vi "temp_dependent_eV-V_slope.vi"() -> ()   [LabVIEW 2016]
uses:
  <vilib>/Analysis/baseanly.llb/Mean (DBL).vi
  <vilib>/Analysis/NI_AALBase.lvlib
  <vilib>/Analysis/NI_AALPro.lvlib
panel:
  out "1/x ( eV/V)":dbl
  out "intercept":dbl
  out "slope (V/eV)":dbl
  out "XY Graph":cluster{dbl[], dbl[]}(graph)
  out "Array 3":dbl[](array[numeric])
  out "Waveform Graph":dbl[][](graph)
  in  "Array 2":i32[](array[numeric])
  out "Array":dbl[][](array[numeric])
  in  "SuperFolder":path=path "B:/SketchSET/SA03008H.20180718/08-BG_Sweep_-5to5_0.1_@0.1Hz"
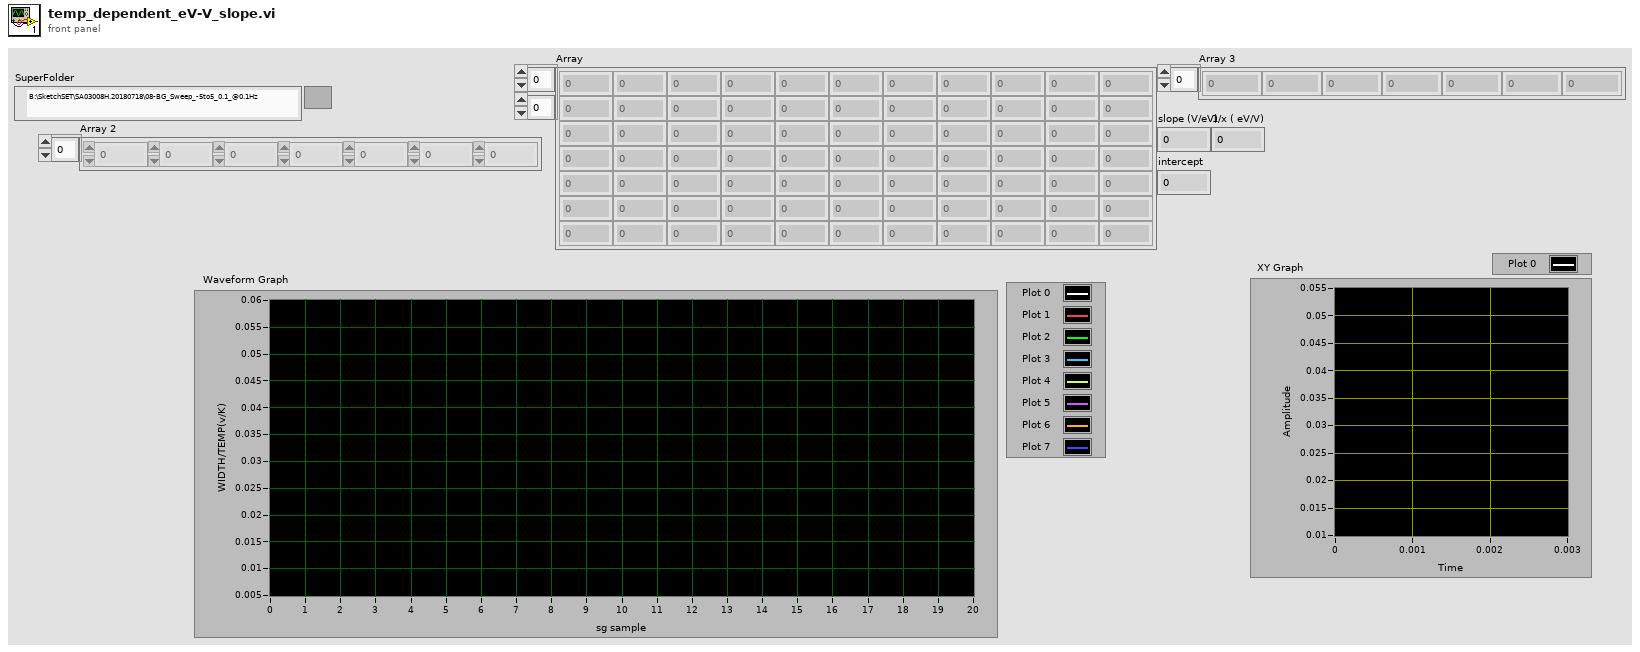
[diagram p1: front panel]
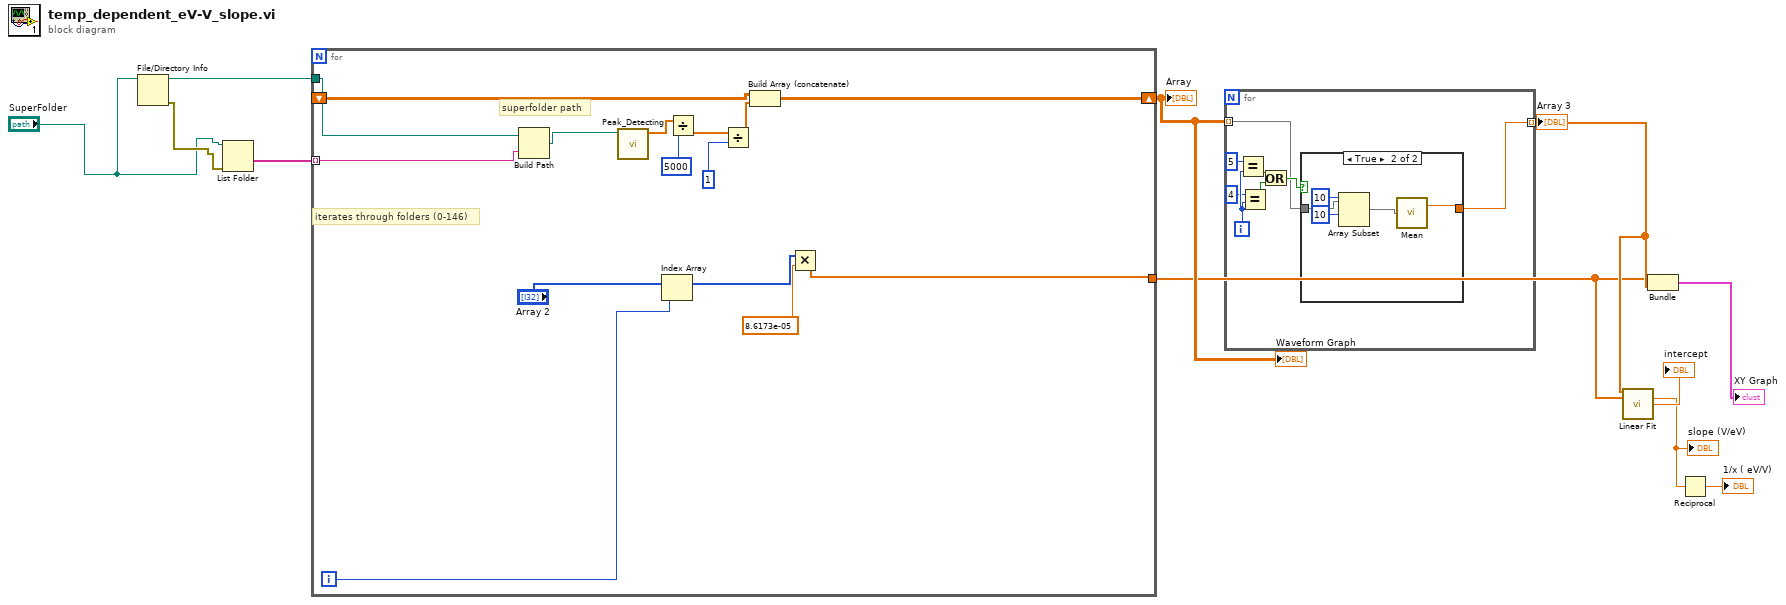
[diagram p0: block diagram]
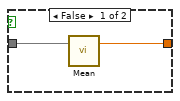
[diagram p2: hidden frame]
diagram:
  n1 = File/Directory Info(path="SuperFolder") -> (path out=w9:path, error out=w11:errorcluster)  [unwired: 1 in, 5 out]
  n2 = List Folder(path="SuperFolder", error in=w11) -> (folder names=w8:string[])  [unwired: 2 in, 3 out]
  n3 = for {
    tunnel: w9 -> [w24]
    tunnel: w8 -> [w25] mode=indexing
    shift-right: [w21] -> w7
    shift-left: _ -> [w20]
    tunnel: [w14] -> w4
    i -> [w19]
    # "iterates through folders (0-146)"
    # "superfolder path"
    n4 = Build Path(base path=w24, name or relative path=w25) -> (appended path=w23:path)
    n5 = call "Peak_Detecting.vi"("Folder or File"=w23) -> ("avg FWHM"=w22:dbl[])  [unwired: 9 in, 1 out]
    n6 = Index Array(array="Array 2", index=w19) -> ()  [unwired: 1 out]
    n7 = Divide(x=w22, y=5000) -> (x/y=w18:dbl[])
    n8 = Divide(x=w18, y=1) -> (x/y=w16:dbl[])
    n9 = Build Array (concatenate)(w20, w16) -> (w21:dbl[][])
    n10 = Multiply(x="Array 2", y=8.6173e-05) -> (x*y=w14:dbl[])
  }
  "Array" <- w7
  "Waveform Graph" <- w7
  n11 = for {
    tunnel: w7 -> [w27] mode=indexing
    tunnel: [w26] -> w5 mode=indexing
    i -> [w33]
    n12 = Equal?(x=5, y=w33) -> (x = y?=w30:bool)
    n13 = Equal?(x=4, y=w33) -> (x = y?=w29:bool)
    n14 = Or(x=w30, y=w29) -> (x .or. y?=w28:bool)
    n15 = case shown="True" w28 {
      tunnel: w27 -> [w35 w40]
      tunnel: [w34 w36] -> w26
      frame False {
        n16 = call-poly <vilib>:"Mean.vi"("X"=w35) -> ("mean"=w34:dbl)  [unwired: 1 out]
      }
      frame True {
        n17 = Array Subset(array=w40, index=10, length=10) -> (w37:dbl[])
        n18 = call-poly <vilib>:"Mean.vi"("X"=w37) -> ("mean"=w36:dbl)  [unwired: 1 out]
      }
    }
  }
  "Array 3" <- w5
  n19 = call <vilib>:"Linear Fit.vi"("Y"=w5, "X"=w4) -> ("slope"=w2:dbl, "intercept"=→"intercept":dbl)  [unwired: 9 in, 3 out]
  "slope (V/eV)" <- w2
  n20 = Bundle(w4, w5) -> (→"XY Graph":cluster{dbl[], dbl[]})  [unwired: 1 in]
  n21 = Reciprocal(x=w2) -> (1/x=→"1/x ( eV/V)":dbl)
